vi "disableAutoRecovery.vi"   [LabVIEW 2015]
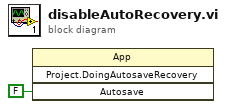
[diagram p0: block diagram]
diagram:
  n1 = invoke class="App" method="Project.DoingAutosaveRecovery"("Autosave"=FALSE ("Auto Save")) -> ()  [unwired: 3 in, 4 out]
